vi "HandleObservationSync.vi"(8 "error in (no error)":errorcluster, 11 "S4GUI in":refnum<class "S4GUI.lvclass">) -> (0 "error out":errorcluster, 3 "S4GUI out":refnum<class "S4GUI.lvclass">)   [LabVIEW 2018, in "S4GUI.lvclass"] (continued)
            tunnel: w4130 -> [w4184 _]
            tunnel: w4124 -> [w4182 _]
            frame False {
              n1516 = case shown="0, Default" w4182 {
                selector: w4182 -> [_ w4199]
                tunnel: [w4186 w4194] -> w4183
                tunnel: w4185 -> [w4189 w4200]
                tunnel: w4184 -> [w4188 _]
                frame 0, Default {
                  n1517 = disable-structure shown="Enabled" {
                    disable-tunnel: w4188 -> [w4191 w4192]
                    disable-tunnel: [w4190 w4192] -> w4187
                    frame Disabled {
                      # "Verifica o incremento \ndo CyclesDone simultaneamente"
                      n1518 = Increment(x=w4191) -> (x+1=w4190:u32)
                    }
                    frame Enabled {
                      # "OV20241106:\nNão verifica mais o CyclesDone\nem 327 enquanto espera o ACTIVE\nem 326."
                    }
                  }
                  n1519 = Bundle By Name(cluster=w4189, "Obs_state"=w4187) -> (w4186:refnum<class "S4GUI.lvclass">)
                }
                frame 1..15 {
                  n1520 = Number To Decimal String(number=w4199) -> (decimal integer string=w4196:string)  [unwired: 1 in]
                  n1521 = Concatenate Strings("CHANNEL ERROR <", w4196, ">: Error flag TRUE - see ACS panel.  HandleObservationSync.vi - state 326.") -> (w4198:string)
                  n1522 = Bundle By Name(cluster=w4200, "Obs_state"=u32 1, "Error Msg"=w4198) -> (w4194:refnum<class "S4GUI.lvclass">)
                }
              }
            }
            frame True {
              # "ACTIVE detectado.\nIniciou aquisição..."
              n1523 = Tick Count (ms)() -> (millisecond timer value=w4201:u32)
              n1524 = local write "time307"(w4201) -> ()
              n1525 = Bundle By Name(cluster=w4204, "Obs_state"=u32 328) -> (w4203:refnum<class "S4GUI.lvclass">)
            }
          }
          n1526 = Bundle By Name(cluster=w4129, "mode EXPOSE"=w4132) -> (w4176:refnum<class "S4GUI.lvclass">)
        }
        frame 327 {
          # "T= canais receberam STOP"
          n1527 = Unbundle By Name(w4328) -> ("cyclesDone"=w4323:u32)
          n1528 = call-dynamic "Read AcquisitionA.vi"("error in (no error)"=w4361, "S4ACS_GUI in"=w4328) -> ("error out"=w4343:errorcluster, "Acquisition.lvclass"=w4344:refnum<class "Acquisition.lvclass">, "S4ACS_GUI out"=w4363:refnum<class "S4GUI.lvclass">)  [unwired: 7 in]
          n1529 = call-dynamic "Read enabled.vi"("error in (no error)"=w4343, "Server in"=w4344) -> ("error out"=w4342:errorcluster, "enabled"=w4319:bool, "Server out"=w4341:refnum<class "Acquisition.lvclass">)  [unwired: 7 in]
          n1530 = case shown="True" w4319 {
            tunnel: w4342 -> [w4517 w4534]
            tunnel: [w4518 w4532] -> w4364
            tunnel: [w4517 w4531] -> w4362
            tunnel: [0 ("State") w4527] -> w4314
            tunnel: w4341 -> [w4518 w4526]
            tunnel: w4323 -> [_ w4525]
            tunnel: [TRUE w4524] -> w4327
            tunnel: [FALSE ("stopping") w4520] -> w4310
            frame False {
            }
            frame True {
              n1531 = call-dynamic "Read Channel.vi"("error in (no error)"=w4534, "Acquisition in"=w4526) -> ("error out"=w4530:errorcluster, "Channel.lvclass"=w4529:refnum<class "Channel.lvclass">, "Acquisition out"=w4533:refnum<class "Acquisition.lvclass">)  [unwired: 7 in]
              n1532 = call-dynamic "Read CyclesDone.vi"("error in (no error)"=w4530, "Channel in"=w4529) -> ("error out"=w4522:errorcluster, "CyclesDone"=w4527:u32, "Channel out"=w4528:refnum<class "Channel.lvclass">)  [unwired: 7 in]
              n1533 = Increment(x=w4525) -> (x+1=w4519:u32)
              n1534 = Equal?(x=w4527, y=w4519) -> (x = y?=w4524:bool)
              n1535 = call-dynamic "Read stopping.vi"("error in (no error)"=w4522, "Channel in"=w4528) -> ("error out"=w4521:errorcluster, "stopping"=w4520:bool, "Channel out"=w4523:refnum<class "Channel.lvclass">)  [unwired: 7 in]
              n1536 = call-dynamic "Write Channel.vi"("error in (no error)"=w4521, "Channel.lvclass"=w4523, "Acquisition in"=w4533) -> ("error out"=w4531:errorcluster, "Acquisition out"=w4532:refnum<class "Acquisition.lvclass">)  [unwired: 7 in]
            }
          }
          n1537 = call-dynamic "Write AcquisitionA.vi"("error in (no error)"=w4362, "Acquisition.lvclass"=w4364, "S4ACS_GUI in"=w4363) -> ("error out"=w4359:errorcluster, "S4ACS_GUI out"=w4358:refnum<class "S4GUI.lvclass">)  [unwired: 7 in]
          n1538 = call "Read AcquisitionB.vi"("error in (no error)"=w4359, "S4ACS_GUI in"=w4358) -> ("error out"=w4337:errorcluster, "Acquisition.lvclass"=w4340:refnum<class "Acquisition.lvclass">, "S4ACS_GUI out"=w4360:refnum<class "S4GUI.lvclass">)  [unwired: 7 in]
          n1539 = call-dynamic "Read enabled.vi"("error in (no error)"=w4337, "Server in"=w4340) -> ("error out"=w4338:errorcluster, "enabled"=w4318:bool, "Server out"=w4339:refnum<class "Acquisition.lvclass">)  [unwired: 7 in]
          n1540 = case shown="True" w4318 {
            tunnel: w4338 -> [w4496 w4513]
            tunnel: w4339 -> [w4497 w4512]
            tunnel: [0 ("State") w4505] -> w4313
            tunnel: [w4496 w4511] -> w4357
            tunnel: [w4497 w4510] -> w4356
            tunnel: w4323 -> [_ w4504]
            tunnel: [TRUE w4503] -> w4324
            tunnel: [FALSE ("stopping") w4499] -> w4309
            frame False {
            }
            frame True {
              n1541 = call-dynamic "Read Channel.vi"("error in (no error)"=w4513, "Acquisition in"=w4512) -> ("error out"=w4508:errorcluster, "Channel.lvclass"=w4509:refnum<class "Channel.lvclass">, "Acquisition out"=w4506:refnum<class "Acquisition.lvclass">)  [unwired: 7 in]
              n1542 = call-dynamic "Read CyclesDone.vi"("error in (no error)"=w4508, "Channel in"=w4509) -> ("error out"=w4501:errorcluster, "CyclesDone"=w4505:u32, "Channel out"=w4507:refnum<class "Channel.lvclass">)  [unwired: 7 in]
              n1543 = Increment(x=w4504) -> (x+1=w4498:u32)
              n1544 = Equal?(x=w4505, y=w4498) -> (x = y?=w4503:bool)
              n1545 = call-dynamic "Read stopping.vi"("error in (no error)"=w4501, "Channel in"=w4507) -> ("error out"=w4500:errorcluster, "stopping"=w4499:bool, "Channel out"=w4502:refnum<class "Channel.lvclass">)  [unwired: 7 in]
              n1546 = call-dynamic "Write Channel.vi"("error in (no error)"=w4500, "Channel.lvclass"=w4502, "Acquisition in"=w4506) -> ("error out"=w4511:errorcluster, "Acquisition out"=w4510:refnum<class "Acquisition.lvclass">)  [unwired: 7 in]
            }
          }
          n1547 = Max & Min(x=w4314, y=w4313) -> (max(x,y)=w4326:u32)  [unwired: 1 out]
          n1548 = call "Write AcquisitionB.vi"("error in (no error)"=w4357, "Acquisition.lvclass"=w4356, "S4ACS_GUI in"=w4360) -> ("error out"=w4349:errorcluster, "S4ACS_GUI out"=w4348:refnum<class "S4GUI.lvclass">)  [unwired: 7 in]
          n1549 = call-dynamic "Read AcquisitionC.vi"("error in (no error)"=w4349, "S4ACS_GUI in"=w4348) -> ("error out"=w4334:errorcluster, "Acquisition.lvclass"=w4336:refnum<class "Acquisition.lvclass">, "S4ACS_GUI out"=w4351:refnum<class "S4GUI.lvclass">)  [unwired: 7 in]
          n1550 = call-dynamic "Read enabled.vi"("error in (no error)"=w4334, "Server in"=w4336) -> ("error out"=w4333:errorcluster, "enabled"=w4317:bool, "Server out"=w4335:refnum<class "Acquisition.lvclass">)  [unwired: 7 in]
          n1551 = case shown="True" w4317 {
            tunnel: [w4475 w4492] -> w4352
            tunnel: [w4476 w4491] -> w4350
            tunnel: w4333 -> [w4475 w4488]
            tunnel: w4335 -> [w4476 w4489]
            tunnel: [0 ("State") w4487] -> w4312
            tunnel: w4323 -> [_ w4486]
            tunnel: [TRUE w4485] -> w4322
            tunnel: [FALSE ("stopping") w4478] -> w4308
            frame False {
            }
            frame True {
              n1552 = call-dynamic "Read Channel.vi"("error in (no error)"=w4488, "Acquisition in"=w4489) -> ("error out"=w4484:errorcluster, "Channel.lvclass"=w4483:refnum<class "Channel.lvclass">, "Acquisition out"=w4490:refnum<class "Acquisition.lvclass">)  [unwired: 7 in]
              n1553 = call-dynamic "Read CyclesDone.vi"("error in (no error)"=w4484, "Channel in"=w4483) -> ("error out"=w4480:errorcluster, "CyclesDone"=w4487:u32, "Channel out"=w4482:refnum<class "Channel.lvclass">)  [unwired: 7 in]
              n1554 = Increment(x=w4486) -> (x+1=w4477:u32)
              n1555 = Equal?(x=w4487, y=w4477) -> (x = y?=w4485:bool)
              n1556 = call-dynamic "Read stopping.vi"("error in (no error)"=w4480, "Channel in"=w4482) -> ("error out"=w4479:errorcluster, "stopping"=w4478:bool, "Channel out"=w4481:refnum<class "Channel.lvclass">)  [unwired: 7 in]
              n1557 = call-dynamic "Write Channel.vi"("error in (no error)"=w4479, "Channel.lvclass"=w4481, "Acquisition in"=w4490) -> ("error out"=w4492:errorcluster, "Acquisition out"=w4491:refnum<class "Acquisition.lvclass">)  [unwired: 7 in]
            }
          }
          n1558 = call-dynamic "Write AcquisitionC.vi"("error in (no error)"=w4352, "Acquisition.lvclass"=w4350, "S4ACS_GUI in"=w4351) -> ("error out"=w4346:errorcluster, "S4ACS_GUI out"=w4347:refnum<class "S4GUI.lvclass">)  [unwired: 7 in]
          n1559 = call-dynamic "Read AcquisitionD.vi"("error in (no error)"=w4346, "S4ACS_GUI in"=w4347) -> ("error out"=w4330:errorcluster, "Acquisition.lvclass"=w4332:refnum<class "Acquisition.lvclass">, "S4ACS_GUI out"=w4353:refnum<class "S4GUI.lvclass">)  [unwired: 7 in]
          n1560 = call-dynamic "Read enabled.vi"("error in (no error)"=w4330, "Server in"=w4332) -> ("error out"=w4329:errorcluster, "enabled"=w4320:bool, "Server out"=w4331:refnum<class "Acquisition.lvclass">)  [unwired: 7 in]
          n1561 = case shown="True" w4320 {
            tunnel: [w4455 w4471] -> w4355
            tunnel: [w4454 w4470] -> w4354
            tunnel: w4331 -> [w4455 w4469]
            tunnel: w4329 -> [w4454 w4468]
            tunnel: [0 ("State") w4466] -> w4311
            tunnel: w4323 -> [_ w4465]
            tunnel: [TRUE w4464] -> w4321
            tunnel: [FALSE ("stopping") w4457] -> w4307
            frame False {
            }
            frame True {
              n1562 = call-dynamic "Read Channel.vi"("error in (no error)"=w4468, "Acquisition in"=w4469) -> ("error out"=w4463:errorcluster, "Channel.lvclass"=w4462:refnum<class "Channel.lvclass">, "Acquisition out"=w4467:refnum<class "Acquisition.lvclass">)  [unwired: 7 in]
              n1563 = call-dynamic "Read CyclesDone.vi"("error in (no error)"=w4463, "Channel in"=w4462) -> ("error out"=w4459:errorcluster, "CyclesDone"=w4466:u32, "Channel out"=w4461:refnum<class "Channel.lvclass">)  [unwired: 7 in]
              n1564 = Increment(x=w4465) -> (x+1=w4456:u32)
              n1565 = Equal?(x=w4466, y=w4456) -> (x = y?=w4464:bool)
              n1566 = call-dynamic "Read stopping.vi"("error in (no error)"=w4459, "Channel in"=w4461) -> ("error out"=w4458:errorcluster, "stopping"=w4457:bool, "Channel out"=w4460:refnum<class "Channel.lvclass">)  [unwired: 7 in]
              n1567 = call-dynamic "Write Channel.vi"("error in (no error)"=w4458, "Channel.lvclass"=w4460, "Acquisition in"=w4467) -> ("error out"=w4470:errorcluster, "Acquisition out"=w4471:refnum<class "Acquisition.lvclass">)  [unwired: 7 in]
            }
          }
          n1568 = Build Array(w4319, w4318, w4317, w4320) -> (w4316:bool[])
          n1569 = Boolean Array To Number(Boolean array=w4316) -> (number=w4315:u32)
          n1570 = Max & Min(x=w4312, y=w4311) -> (max(x,y)=w4325:u32)  [unwired: 1 out]
          n1571 = Compound Arithmetic op=AND(w4327, w4324, w4322, w4321) -> (w4306:bool)
          n1572 = case shown="15" w4315 {
            tunnel: w4314 -> [w4407 _ w4419 _ w4428 _ w4434 w4440 _ w4446 w4449 _]
            tunnel: w4311 -> [w4406 w4410 w4415 w4422 w4423 w4431 w4433 _ _ _ _ _]
            tunnel: w4313 -> [w4405 w4408 _ _ w4427 w4429 _ w4439 w4443 _ w4448 _]
            tunnel: w4312 -> [w4404 w4409 w4414 w4420 _ _ _ w4438 w4442 w4445 _ _]
            tunnel: [w4400 w4411 w4416 w4421 w4424 w4430 w4432 w4435 w4441 w4444 w4447 TRUE] -> _
            frame 15 {
              # "A,B,C,D ativos"
              n1573 = Equal?(x=w4407, y=w4405) -> (x = y?=w4403:bool)
              n1574 = Equal?(x=w4404, y=w4406) -> (x = y?=w4401:bool)
              n1575 = Equal?(x=w4405, y=w4404) -> (x = y?=w4402:bool)
              n1576 = Compound Arithmetic op=AND(w4403, w4402, w4401) -> (w4400:bool)
            }
            frame 14 {
              # "B,C e,D ativos"
              n1577 = Equal?(x=w4408, y=w4409) -> (x = y?=w4413:bool)
              n1578 = Equal?(x=w4409, y=w4410) -> (x = y?=w4412:bool)
              n1579 = Compound Arithmetic op=AND(w4413, w4412) -> (w4411:bool)
            }
            frame 13 {
              # "A,C e,D ativos"
              n1580 = Equal?(x=w4419, y=w4414) -> (x = y?=w4418:bool)
              n1581 = Equal?(x=w4414, y=w4415) -> (x = y?=w4417:bool)
              n1582 = Compound Arithmetic op=AND(w4418, w4417) -> (w4416:bool)
            }
            frame 12 {
              # "Só C e D ativos"
              n1583 = Equal?(x=w4420, y=w4422) -> (x = y?=w4421:bool)
            }
            frame 11 {
              # "A,B e,D ativos"
              n1584 = Equal?(x=w4428, y=w4427) -> (x = y?=w4426:bool)
              n1585 = Equal?(x=w4427, y=w4423) -> (x = y?=w4425:bool)
              n1586 = Compound Arithmetic op=AND(w4426, w4425) -> (w4424:bool)
            }
            frame 10 {
              # "Só B e D ativos"
              n1587 = Equal?(x=w4429, y=w4431) -> (x = y?=w4430:bool)
            }
            frame 9 {
              # "Só A e D ativos"
              n1588 = Equal?(x=w4434, y=w4433) -> (x = y?=w4432:bool)
            }
            frame 7 {
              # "A,B,C ativos"
              n1589 = Equal?(x=w4440, y=w4439) -> (x = y?=w4437:bool)
              n1590 = Equal?(x=w4439, y=w4438) -> (x = y?=w4436:bool)
              n1591 = Compound Arithmetic op=AND(w4437, w4436) -> (w4435:bool)
            }
            frame 6 {
              # "Só B e C ativos"
              n1592 = Equal?(x=w4443, y=w4442) -> (x = y?=w4441:bool)
            }
            frame 5 {
              # "Só A e C ativos"
              n1593 = Equal?(x=w4446, y=w4445) -> (x = y?=w4444:bool)
            }
            frame 3 {
              # "só A e B ativos"
              n1594 = Equal?(x=w4449, y=w4448) -> (x = y?=w4447:bool)
            }
            frame 0..2, 4, 8, Default {
              # "nenhum ou só 1  \ncanal ativo."
            }
          }
          n1595 = Max & Min(x=w4326, y=w4325) -> (max(x,y)=w4304:u32)  [unwired: 1 out]
          n1596 = Compound Arithmetic op=OR(w4310, w4309, w4308, w4307) -> (w4305:bool)
          n1597 = call-dynamic "Write AcquisitionD.vi"("error in (no error)"=w4354, "Acquisition.lvclass"=w4355, "S4ACS_GUI in"=w4353) -> ("error out"=w4345:errorcluster, "S4ACS_GUI out"=w4302:refnum<class "S4GUI.lvclass">)  [unwired: 7 in]
          n1598 = case shown="False" w4306 {
            tunnel: w4302 -> [w4367 w4388]
            tunnel: [w4373 w4387] -> w4301
            tunnel: w4305 -> [_ w4389]
            tunnel: w4304 -> [_ w4386]
            tunnel: w4303 -> [w4365 w4385]
            frame False {
              # "Aguardando iniciar exposição por 5s"
              n1599 = local read "time1"() -> (w4366:u32)
              n1600 = Tick Count (ms)() -> (millisecond timer value=w4372:u32)
              n1601 = Subtract(x=w4372, y=w4366) -> (x-y=w4369:u32)
              n1602 = To Double Precision Float(number=w4369) -> (double precision float=w4371:dbl)
              n1603 = Less?(x=5000.0 ("y"), y=w4371) -> (x < y?=w4370:bool)
              n1604 = case shown="True" w4370 {
                tunnel: w4367 -> [w4377 w4384]
                tunnel: [w4376 w4383] -> w4373
                tunnel: w4365 -> [w4375 _]
                frame False {
                  n1605 = disable-structure shown="Enabled" {
                    disable-tunnel: w4375 -> [w4379 w4380]
                    disable-tunnel: [w4378 w4380] -> w4374
                    frame Disabled {
                      # "Volta para esperar ACTIVE."
                      n1606 = Decrement(x=w4379) -> (x-1=w4378:u32)
                    }
                    frame Enabled {
                    }
                  }
                  n1607 = Bundle By Name(cluster=w4377, "Obs_state"=w4374) -> (w4376:refnum<class "S4GUI.lvclass">)
                }
                frame True {
                  n1608 = Bundle By Name(cluster=w4384, "Obs_state"=u32 1, "Error Msg"="ERROR: Init Acquisition Timeout. HandleObservationSync.vi - state 327.") -> (w4383:refnum<class "S4GUI.lvclass">)
                }
              }
            }
            frame True {
              # "STOP?"
              # "CIclo Avançou."
              n1609 = case shown="False" w4389 {
                tunnel: w4388 -> [w4393 w4399]
                tunnel: [w4392 w4398] -> w4387
                tunnel: w4386 -> [w4391 w4397]
                tunnel: w4385 -> [_ w4396]
                frame True {
                  # "STOP acionado."
                  n1610 = Bundle By Name(cluster=w4393, "Obs_state"=u32 0, "cyclesDone"=w4391) -> (w4392:refnum<class "S4GUI.lvclass">)
                }
                frame False {
                  # "Vai verificar fim dos ciclos"
                  n1611 = Increment(x=w4396) -> (x+1=w4395:u32)
                  n1612 = Increment(x=w4395) -> (x+1=w4394:u32)
                  n1613 = Bundle By Name(cluster=w4399, "Obs_state"=w4394, "cyclesDone"=w4397) -> (w4398:refnum<class "S4GUI.lvclass">)
                }
              }
            }
          }
        }
        frame 328 {
          # "T= canais receberam STOP"
          n1614 = Unbundle By Name(w4559) -> ("cyclesDone"=w4553:u32)
          n1615 = call-dynamic "Read AcquisitionA.vi"("error in (no error)"=w4595, "S4ACS_GUI in"=w4559) -> ("error out"=w4574:errorcluster, "Acquisition.lvclass"=w4575:refnum<class "Acquisition.lvclass">, "S4ACS_GUI out"=w4597:refnum<class "S4GUI.lvclass">)  [unwired: 7 in]
          n1616 = call-dynamic "Read enabled.vi"("error in (no error)"=w4574, "Server in"=w4575) -> ("error out"=w4573:errorcluster, "enabled"=w4549:bool, "Server out"=w4572:refnum<class "Acquisition.lvclass">)  [unwired: 7 in]
          n1617 = case shown="False" w4549 {
            tunnel: w4573 -> [w4746 w4763]
            tunnel: [w4747 w4761] -> w4598
            tunnel: [w4746 w4760] -> w4596
            tunnel: [0 ("State") w4756] -> w4544
            tunnel: w4572 -> [w4747 w4755]
            tunnel: w4553 -> [_ w4754]
            tunnel: [TRUE w4753] -> w4558
            tunnel: [FALSE ("stopping") w4749] -> w4540
            frame False {
            }
            frame True {
              n1618 = call-dynamic "Read Channel.vi"("error in (no error)"=w4763, "Acquisition in"=w4755) -> ("error out"=w4759:errorcluster, "Channel.lvclass"=w4758:refnum<class "Channel.lvclass">, "Acquisition out"=w4762:refnum<class "Acquisition.lvclass">)  [unwired: 7 in]
              n1619 = call-dynamic "Read CyclesDone.vi"("error in (no error)"=w4759, "Channel in"=w4758) -> ("error out"=w4751:errorcluster, "CyclesDone"=w4756:u32, "Channel out"=w4757:refnum<class "Channel.lvclass">)  [unwired: 7 in]
              n1620 = Increment(x=w4754) -> (x+1=w4748:u32)
              n1621 = Equal?(x=w4756, y=w4748) -> (x = y?=w4753:bool)
              n1622 = call-dynamic "Read stopping.vi"("error in (no error)"=w4751, "Channel in"=w4757) -> ("error out"=w4750:errorcluster, "stopping"=w4749:bool, "Channel out"=w4752:refnum<class "Channel.lvclass">)  [unwired: 7 in]
              n1623 = call-dynamic "Write Channel.vi"("error in (no error)"=w4750, "Channel.lvclass"=w4752, "Acquisition in"=w4762) -> ("error out"=w4760:errorcluster, "Acquisition out"=w4761:refnum<class "Acquisition.lvclass">)  [unwired: 7 in]
            }
          }
          n1624 = call-dynamic "Write AcquisitionA.vi"("error in (no error)"=w4596, "Acquisition.lvclass"=w4598, "S4ACS_GUI in"=w4597) -> ("error out"=w4591:errorcluster, "S4ACS_GUI out"=w4590:refnum<class "S4GUI.lvclass">)  [unwired: 7 in]
          n1625 = call "Read AcquisitionB.vi"("error in (no error)"=w4591, "S4ACS_GUI in"=w4590) -> ("error out"=w4568:errorcluster, "Acquisition.lvclass"=w4571:refnum<class "Acquisition.lvclass">, "S4ACS_GUI out"=w4592:refnum<class "S4GUI.lvclass">)  [unwired: 7 in]
          n1626 = call-dynamic "Read enabled.vi"("error in (no error)"=w4568, "Server in"=w4571) -> ("error out"=w4569:errorcluster, "enabled"=w4548:bool, "Server out"=w4570:refnum<class "Acquisition.lvclass">)  [unwired: 7 in]
          n1627 = case shown="True" w4548 {
            tunnel: w4569 -> [w4725 w4742]
            tunnel: w4570 -> [w4726 w4741]
            tunnel: [0 ("State") w4734] -> w4543
            tunnel: [w4725 w4740] -> w4589
            tunnel: [w4726 w4739] -> w4588
            tunnel: w4553 -> [_ w4733]
            tunnel: [TRUE w4732] -> w4554
            tunnel: [FALSE ("stopping") w4728] -> w4539
            frame False {
            }
            frame True {
              n1628 = call-dynamic "Read Channel.vi"("error in (no error)"=w4742, "Acquisition in"=w4741) -> ("error out"=w4737:errorcluster, "Channel.lvclass"=w4738:refnum<class "Channel.lvclass">, "Acquisition out"=w4735:refnum<class "Acquisition.lvclass">)  [unwired: 7 in]
              n1629 = call-dynamic "Read CyclesDone.vi"("error in (no error)"=w4737, "Channel in"=w4738) -> ("error out"=w4730:errorcluster, "CyclesDone"=w4734:u32, "Channel out"=w4736:refnum<class "Channel.lvclass">)  [unwired: 7 in]
              n1630 = Increment(x=w4733) -> (x+1=w4727:u32)
              n1631 = Equal?(x=w4734, y=w4727) -> (x = y?=w4732:bool)
              n1632 = call-dynamic "Read stopping.vi"("error in (no error)"=w4730, "Channel in"=w4736) -> ("error out"=w4729:errorcluster, "stopping"=w4728:bool, "Channel out"=w4731:refnum<class "Channel.lvclass">)  [unwired: 7 in]
              n1633 = call-dynamic "Write Channel.vi"("error in (no error)"=w4729, "Channel.lvclass"=w4731, "Acquisition in"=w4735) -> ("error out"=w4740:errorcluster, "Acquisition out"=w4739:refnum<class "Acquisition.lvclass">)  [unwired: 7 in]
            }
          }
          n1634 = Max & Min(x=w4544, y=w4543) -> (max(x,y)=w4557:u32)  [unwired: 1 out]
          n1635 = call "Write AcquisitionB.vi"("error in (no error)"=w4589, "Acquisition.lvclass"=w4588, "S4ACS_GUI in"=w4592) -> ("error out"=w4581:errorcluster, "S4ACS_GUI out"=w4580:refnum<class "S4GUI.lvclass">)  [unwired: 7 in]
          n1636 = call-dynamic "Read AcquisitionC.vi"("error in (no error)"=w4581, "S4ACS_GUI in"=w4580) -> ("error out"=w4565:errorcluster, "Acquisition.lvclass"=w4567:refnum<class "Acquisition.lvclass">, "S4ACS_GUI out"=w4583:refnum<class "S4GUI.lvclass">)  [unwired: 7 in]
          n1637 = call-dynamic "Read enabled.vi"("error in (no error)"=w4565, "Server in"=w4567) -> ("error out"=w4564:errorcluster, "enabled"=w4547:bool, "Server out"=w4566:refnum<class "Acquisition.lvclass">)  [unwired: 7 in]
          n1638 = case shown="False" w4547 {
            tunnel: [w4704 w4721] -> w4584
            tunnel: [w4705 w4720] -> w4582
            tunnel: w4564 -> [w4704 w4717]
            tunnel: w4566 -> [w4705 w4718]
            tunnel: [0 ("State") w4716] -> w4542
            tunnel: w4553 -> [_ w4715]
            tunnel: [TRUE w4714] -> w4552
            tunnel: [FALSE ("stopping") w4707] -> w4538
            frame False {
            }
            frame True {
              n1639 = call-dynamic "Read Channel.vi"("error in (no error)"=w4717, "Acquisition in"=w4718) -> ("error out"=w4713:errorcluster, "Channel.lvclass"=w4712:refnum<class "Channel.lvclass">, "Acquisition out"=w4719:refnum<class "Acquisition.lvclass">)  [unwired: 7 in]
              n1640 = call-dynamic "Read CyclesDone.vi"("error in (no error)"=w4713, "Channel in"=w4712) -> ("error out"=w4709:errorcluster, "CyclesDone"=w4716:u32, "Channel out"=w4711:refnum<class "Channel.lvclass">)  [unwired: 7 in]
              n1641 = Increment(x=w4715) -> (x+1=w4706:u32)
              n1642 = Equal?(x=w4716, y=w4706) -> (x = y?=w4714:bool)
              n1643 = call-dynamic "Read stopping.vi"("error in (no error)"=w4709, "Channel in"=w4711) -> ("error out"=w4708:errorcluster, "stopping"=w4707:bool, "Channel out"=w4710:refnum<class "Channel.lvclass">)  [unwired: 7 in]
              n1644 = call-dynamic "Write Channel.vi"("error in (no error)"=w4708, "Channel.lvclass"=w4710, "Acquisition in"=w4719) -> ("error out"=w4721:errorcluster, "Acquisition out"=w4720:refnum<class "Acquisition.lvclass">)  [unwired: 7 in]
            }
          }
          n1645 = call-dynamic "Write AcquisitionC.vi"("error in (no error)"=w4584, "Acquisition.lvclass"=w4582, "S4ACS_GUI in"=w4583) -> ("error out"=w4578:errorcluster, "S4ACS_GUI out"=w4579:refnum<class "S4GUI.lvclass">)  [unwired: 7 in]
          n1646 = call-dynamic "Read AcquisitionD.vi"("error in (no error)"=w4578, "S4ACS_GUI in"=w4579) -> ("error out"=w4561:errorcluster, "Acquisition.lvclass"=w4563:refnum<class "Acquisition.lvclass">, "S4ACS_GUI out"=w4585:refnum<class "S4GUI.lvclass">)  [unwired: 7 in]
          n1647 = call-dynamic "Read enabled.vi"("error in (no error)"=w4561, "Server in"=w4563) -> ("error out"=w4560:errorcluster, "enabled"=w4550:bool, "Server out"=w4562:refnum<class "Acquisition.lvclass">)  [unwired: 7 in]
          n1648 = case shown="True" w4550 {
            tunnel: [w4684 w4700] -> w4587
            tunnel: [w4683 w4699] -> w4586
            tunnel: w4562 -> [w4684 w4698]
            tunnel: w4560 -> [w4683 w4697]
            tunnel: [0 ("State") w4695] -> w4541
            tunnel: w4553 -> [_ w4694]
            tunnel: [TRUE w4693] -> w4551
            tunnel: [FALSE ("stopping") w4686] -> w4537
            frame False {
            }
            frame True {
              n1649 = call-dynamic "Read Channel.vi"("error in (no error)"=w4697, "Acquisition in"=w4698) -> ("error out"=w4692:errorcluster, "Channel.lvclass"=w4691:refnum<class "Channel.lvclass">, "Acquisition out"=w4696:refnum<class "Acquisition.lvclass">)  [unwired: 7 in]
              n1650 = call-dynamic "Read CyclesDone.vi"("error in (no error)"=w4692, "Channel in"=w4691) -> ("error out"=w4688:errorcluster, "CyclesDone"=w4695:u32, "Channel out"=w4690:refnum<class "Channel.lvclass">)  [unwired: 7 in]
              n1651 = Increment(x=w4694) -> (x+1=w4685:u32)
              n1652 = Equal?(x=w4695, y=w4685) -> (x = y?=w4693:bool)
              n1653 = call-dynamic "Read stopping.vi"("error in (no error)"=w4688, "Channel in"=w4690) -> ("error out"=w4687:errorcluster, "stopping"=w4686:bool, "Channel out"=w4689:refnum<class "Channel.lvclass">)  [unwired: 7 in]
              n1654 = call-dynamic "Write Channel.vi"("error in (no error)"=w4687, "Channel.lvclass"=w4689, "Acquisition in"=w4696) -> ("error out"=w4699:errorcluster, "Acquisition out"=w4700:refnum<class "Acquisition.lvclass">)  [unwired: 7 in]
            }
          }
          n1655 = Build Array(w4549, w4548, w4547, w4550) -> (w4546:bool[])
          n1656 = Boolean Array To Number(Boolean array=w4546) -> (number=w4545:u32)
          n1657 = Max & Min(x=w4542, y=w4541) -> (max(x,y)=w4556:u32)  [unwired: 1 out]
          n1658 = Compound Arithmetic op=AND(w4558, w4554, w4552, w4551) -> (w4535:bool)
          n1659 = case shown="15" w4545 {
            tunnel: w4544 -> [w4606 _ w4618 _ w4627 _ w4633 w4639 _ w4645 w4648 _]
            tunnel: w4541 -> [w4605 w4609 w4614 w4621 w4622 w4630 w4632 _ _ _ _ _]
            tunnel: w4543 -> [w4604 w4607 _ _ w4626 w4628 _ w4638 w4642 _ w4647 _]
            tunnel: w4542 -> [w4603 w4608 w4613 w4619 _ _ _ w4637 w4641 w4644 _ _]
            tunnel: [w4599 w4610 w4615 w4620 w4623 w4629 w4631 w4634 w4640 w4643 w4646 TRUE] -> _
            frame 15 {
              # "A,B,C,D ativos"
              n1660 = Equal?(x=w4606, y=w4604) -> (x = y?=w4602:bool)
              n1661 = Equal?(x=w4603, y=w4605) -> (x = y?=w4600:bool)
              n1662 = Equal?(x=w4604, y=w4603) -> (x = y?=w4601:bool)
              n1663 = Compound Arithmetic op=AND(w4602, w4601, w4600) -> (w4599:bool)
            }
            frame 14 {
              # "B,C e,D ativos"
              n1664 = Equal?(x=w4607, y=w4608) -> (x = y?=w4612:bool)
              n1665 = Equal?(x=w4608, y=w4609) -> (x = y?=w4611:bool)
              n1666 = Compound Arithmetic op=AND(w4612, w4611) -> (w4610:bool)
            }
            frame 13 {
              # "A,C e,D ativos"
              n1667 = Equal?(x=w4618, y=w4613) -> (x = y?=w4617:bool)
              n1668 = Equal?(x=w4613, y=w4614) -> (x = y?=w4616:bool)
              n1669 = Compound Arithmetic op=AND(w4617, w4616) -> (w4615:bool)
            }
            frame 12 {
              # "Só C e D ativos"
              n1670 = Equal?(x=w4619, y=w4621) -> (x = y?=w4620:bool)
            }
            frame 11 {
              # "A,B e,D ativos"
              n1671 = Equal?(x=w4627, y=w4626) -> (x = y?=w4625:bool)
              n1672 = Equal?(x=w4626, y=w4622) -> (x = y?=w4624:bool)
              n1673 = Compound Arithmetic op=AND(w4625, w4624) -> (w4623:bool)
            }
            frame 10 {
              # "Só B e D ativos"
              n1674 = Equal?(x=w4628, y=w4630) -> (x = y?=w4629:bool)
            }
            frame 9 {
              # "Só A e D ativos"
              n1675 = Equal?(x=w4633, y=w4632) -> (x = y?=w4631:bool)
            }
            frame 7 {
              # "A,B,C ativos"
              n1676 = Equal?(x=w4639, y=w4638) -> (x = y?=w4636:bool)
              n1677 = Equal?(x=w4638, y=w4637) -> (x = y?=w4635:bool)
              n1678 = Compound Arithmetic op=AND(w4636, w4635) -> (w4634:bool)
            }
            frame 6 {
              # "Só B e C ativos"
              n1679 = Equal?(x=w4642, y=w4641) -> (x = y?=w4640:bool)
            }
            frame 5 {
              # "Só A e C ativos"
              n1680 = Equal?(x=w4645, y=w4644) -> (x = y?=w4643:bool)
            }
            frame 3 {
              # "só A e B ativos"
              n1681 = Equal?(x=w4648, y=w4647) -> (x = y?=w4646:bool)
            }
            frame 0..2, 4, 8, Default {
              # "nenhum ou só 1  \ncanal ativo."
            }
          }
          n1682 = Max & Min(x=w4557, y=w4556) -> (max(x,y)=w4555:u32)  [unwired: 1 out]
          n1683 = Compound Arithmetic op=OR(w4540, w4539, w4538, w4537) -> (w4536:bool)
          n1684 = call-dynamic "Write AcquisitionD.vi"("error in (no error)"=w4586, "Acquisition.lvclass"=w4587, "S4ACS_GUI in"=w4585) -> ("error out"=w4576:errorcluster, "S4ACS_GUI out"=w4577:refnum<class "S4GUI.lvclass">)  [unwired: 7 in]
          n1685 = case shown="False" w4535 {
            tunnel: w4577 -> [w4660 w4670]
            tunnel: [w4659 w4669] -> w4594
            tunnel: w4593 -> [_ w4668]
            tunnel: w4555 -> [_ w4667]
            tunnel: w4536 -> [_ w4666]
            frame False {
              # "Aguardando avanço do ciclo."
              n1686 = local read "time307"() -> (w4650:u32)
              n1687 = Tick Count (ms)() -> (millisecond timer value=w4658:u32)
              n1688 = Subtract(x=w4658, y=w4650) -> (x-y=w4655:u32)
              n1689 = call-dynamic "GetGreatestCube.vi"("S4GUI in"=w4660) -> ("S4GUI out"=w4651:refnum<class "S4GUI.lvclass">, "greatest (ms)"=w4653:dbl)  [unwired: 8 in, 1 out]
              n1690 = To Double Precision Float(number=w4655) -> (double precision float=w4657:dbl)
              n1691 = Add(x=5000.0 ("y"), y=w4653) -> (x+y=w4652:dbl)
              n1692 = Less?(x=w4652, y=w4657) -> (x < y?=w4656:bool)
              n1693 = case shown="False" w4656 {
                tunnel: w4651 -> [w4661 w4665]
                tunnel: [w4661 w4664] -> w4659
                frame False {
                }
                frame True {
                  n1694 = Bundle By Name(cluster=w4665, "Obs_state"=u32 1, "Error Msg"="ERROR: Acquisition Timeout. HandleObservationSync.vi - state 328.") -> (w4664:refnum<class "S4GUI.lvclass">)
                }
              }
            }
            frame True {
              # "Ciclo avançou."
              # "STOP?"
              n1695 = case shown="False" w4666 {
                tunnel: w4670 -> [w4674 w4679]
                tunnel: [w4673 w4678] -> w4669
                tunnel: w4668 -> [_ w4676]
                tunnel: w4667 -> [w4672 w4675]
                frame True {
                  n1696 = Bundle By Name(cluster=w4674, "Obs_state"=u32 0, "cyclesDone"=w4672) -> (w4673:refnum<class "S4GUI.lvclass">)
                }
                frame False {
                  n1697 = Increment(x=w4676) -> (x+1=w4677:u32)
                  n1698 = Bundle By Name(cluster=w4679, "Obs_state"=w4677, "cyclesDone"=w4675) -> (w4678:refnum<class "S4GUI.lvclass">)
                }
              }
            }
          }
        }
        frame 329 {
          n1699 = disable-structure shown="Enabled" {
            disable-tunnel: w4768 -> [w4782 w4788]
            disable-tunnel: w4767 -> [w4781 w4795]
            disable-tunnel: [w4780 w4795] -> w4766
            disable-tunnel: [w4778 w4796] -> w4765
            disable-tunnel: w4764 -> [_ w4789]
            frame Disabled {
              n1700 = call-dynamic "Read ciclos.vi"("error in (no error)"=w4781, "S4ACS_GUI in"=w4782) -> ("error out"=w4770:errorcluster, "ciclos"=w4775:u32, "S4ACS_GUI out"=w4783:refnum<class "S4GUI.lvclass">)  [unwired: 7 in]
              n1701 = Decrement(x=w4775) -> (x-1=w4769:u32)
              n1702 = Greater Than 0?(x=w4769) -> (x > 0?=w4776:bool)
              n1703 = case shown="False" w4776 {
                selector: w4776 -> [w4785 w4787]
                tunnel: w4769 -> [_ w4786]
                tunnel: [w4785 w4787] -> w4774
                tunnel: [u32 0 w4786] -> w4771
                frame False {
                }
                frame True {
                }
              }
              n1704 = Select(t=u32 323, s=w4774, f=u32 0) -> (s? t:f=w4777:u32)
              n1705 = call-dynamic "Write ciclos.vi"("error in (no error)"=w4770, "ciclos"=w4771, "S4ACS_GUI in"=w4783) -> ("error out"=w4780:errorcluster, "S4ACS_GUI out"=w4779:refnum<class "S4GUI.lvclass">)  [unwired: 7 in]
              n1706 = Bundle By Name(cluster=w4779, "Obs_state"=w4777) -> (w4778:refnum<class "S4GUI.lvclass">)
            }
            frame Enabled {
              n1707 = Unbundle By Name(w4788) -> ("TotalCiclos"=w4798:u32, "cyclesDone"=w4797:u32)
              n1708 = Subtract(x=w4798, y=w4797) -> (x-y=w4791:u32)
              n1709 = Greater Than 0?(x=w4791) -> (x > 0?=w4794:bool)
              n1710 = disable-structure shown="Enabled" {
                disable-tunnel: [w4800 u32 325 ("t")] -> w4790
                disable-tunnel: w4789 -> [w4799 _]
                frame Disabled {
                  n1711 = Increment(x=w4799) -> (x+1=w4800:u32)
                }
                frame Enabled {
                }
              }
              n1712 = Select(t=w4790, s=w4794, f=u32 0) -> (s? t:f=w4793:u32)
              n1713 = Bundle By Name(cluster=w4788, "ciclos"=w4791, "Obs_state"=w4793) -> (w4796:refnum<class "S4GUI.lvclass">)
            }
          }
        }
        frame 350 {
          n1714 = flat-sequence {
            tunnel: w4803 -> [w4843]
            tunnel: [w4843] -> w4802
            frame #0 {
              n1715 = Tick Count (ms)() -> (millisecond timer value=→"timer350":u32)
            }
          }
          n1716 = call "Read Instrument.lvclass.vi"("error in (no error)"=w4802, "S4ACS_GUI in"=w4838) -> ("error out"=w4841:errorcluster, "Instrument.lvclass"=w4842:refnum<class "Instrument.lvclass">, "S4ACS_GUI out"=w4839:refnum<class "S4GUI.lvclass">)  [unwired: 7 in]
          n1717 = call "Read WPROT.vi"("error in (no error)"=w4841, "Instrument in"=w4842) -> ("error out"=w4831:errorcluster, "Opt_Selector.lvclass"=w4832:refnum<class "Opt_Selector.lvclass">, "Instrument out"=w4840:refnum<class "Instrument.lvclass">)  [unwired: 7 in]
          n1718 = call-dynamic "getTargetPos.vi"("error in (no error)"=w4831, "Opt_Selector in"=w4832) -> ("error out"=w4830:errorcluster, "Target Pos"=w4810:u16, "Opt_Selector out"=w4829:refnum<class "Opt_Selector.lvclass">)  [unwired: 7 in]
          n1719 = Build Array(-1.0 ("element"), 0.0 ("element"), 22.5 ("element"), 45.0 ("element"), 67.5 ("element"), 90.0 ("element"), 112.5 ("element"), 135.0 ("element"), 157.5 ("element"), 180.0 ("element"), 202.5 ("element"), 225.0 ("element"), 247.5 ("element"), 270.0 ("element"), 292.5 ("element"), 315.0 ("element"), 337.5 ("element")) -> (w4822:dbl[])
          n1720 = Index Array(array=w4822, index=w4810) -> (element=w4809:dbl)
          n1721 = case shown="0, Default" w4810 {
            selector: w4810 -> [_ w4872]
            tunnel: w4840 -> [w4852 w4860]
            tunnel: [w4852 w4860] -> w4805
            tunnel: [w4849 w4859] -> w4804
            tunnel: w4835 -> [_ w4874]
            tunnel: [u32 352 w4873] -> w4834
            tunnel: w4830 -> [w4850 w4868]
            tunnel: w4829 -> [w4851 w4867]
            tunnel: w4809 -> [_ w4862]
            tunnel: [w4847 w4861] -> w4806
            frame 0, Default {
              # "Terminou uma sequência.\nRecupera as posições em SEQ e desvia para 311 para verificar se há mais ciclos."
              # "Recupera a sequencia anterior para o caso \nde repetição da sequencia (sem precisar clicar \nnas posicoes desejadas novamente)."
              n1722 = call-dynamic "Read sequencia_ant.vi"("error in (no error)"=w4850, "Opt_Selector in"=w4851) -> ("error out"=w4846:errorcluster, "sequencia_ant"=w4845:u16, "Opt_Selector out"=w4848:refnum<class "Opt_Selector.lvclass">)  [unwired: 7 in]
              n1723 = call-dynamic "Write sequencia.vi"("error in (no error)"=w4846, "sequencia"=w4845, "Opt_Selector in"=w4848) -> ("error out"=w4849:errorcluster, "Opt_Selector out"=w4847:refnum<class "Opt_Selector.lvclass">)  [unwired: 7 in]
            }
            frame 1..16 {
              # "Espera até 40 x 0.25s (= 10s) para\nmecanismo entrar em READY"
              n1724 = Number To Decimal String(number=w4872) -> (decimal integer string=w4871:string)  [unwired: 1 in]
              n1725 = Concatenate Strings("WP" ("string"), w4871) -> (w4869:string)
              n1726 = call "Write target name.vi"("error in (no error)"=w4868, "target name"=w4869, "Optics in"=w4867) -> ("error out"=w4865:errorcluster, "Optics out"=w4866:refnum<class "Opt_Selector.lvclass">)  [unwired: 7 in]
              n1727 = call "Write target.vi"("error in (no error)"=w4865, "target"=w4862, "Optics in"=w4866) -> ("error out"=w4864:errorcluster, "Optics out"=w4863:refnum<class "Opt_Selector.lvclass">)  [unwired: 7 in]
              n1728 = call-dynamic "Read State Machine.vi"("error in (no error)"=w4864, "Device in"=w4863) -> ("error out"=w4876:errorcluster, "State Machine.lvclass"=w4878:refnum<class "State Machine.lvclass">, "Device out"=w4875:refnum<class "Opt_Selector.lvclass">)  [unwired: 7 in]
              n1729 = Increment(x=w4874) -> (x+1=w4873:u32)
              n1730 = call "Next State.vi"("error in (no error)"=w4876, "New_State"=1, "State Machine in"=w4878) -> ("error out"=w4856:errorcluster, "State Machine out"=w4858:refnum<class "State Machine.lvclass">)  [unwired: 7 in]
              n1731 = call-dynamic "Write Timer.vi"("error in (no error)"=w4856, "Timer"=u32 40, "State Machine in"=w4858) -> ("error out"=w4855:errorcluster, "State Machine out"=w4857:refnum<class "State Machine.lvclass">)  [unwired: 7 in]
              n1732 = call-dynamic "Write State Machine.vi"("error in (no error)"=w4855, "State Machine.lvclass"=w4857, "Device in"=w4875) -> ("error out"=w4859:errorcluster, "Device out"=w4861:refnum<class "Opt_Selector.lvclass">)  [unwired: 7 in]
            }
          }
          n1733 = call "Write WPROT.vi"("error in (no error)"=w4804, "Opt_Selector.lvclass"=w4806, "Instrument in"=w4805) -> ("error out"=w4808:errorcluster, "Instrument out"=w4807:refnum<class "Instrument.lvclass">)  [unwired: 7 in]
          n1734 = call "Write Instrument.lvclass.vi"("error in (no error)"=w4808, "Instrument.lvclass"=w4807, "S4ACS_GUI in"=w4839) -> ("error out"=w4837:errorcluster, "S4ACS_GUI out"=w4836:refnum<class "S4GUI.lvclass">)  [unwired: 7 in]
          n1735 = Bundle By Name(cluster=w4836, "Obs_state"=w4834) -> (w4833:refnum<class "S4GUI.lvclass">)
        }
        frame 351 {
          # "Espera terminar o movimento da lamina para disparar a aquisição\ndos canais ativos.\n\nOV 20230424: Não precisa mais atualizar o valor de WPPOS com o\ncomando WRITE_HEADER porque o ACS já recebeu a sequência de\nposições da lâmina."
          n1736 = flat-sequence {
            tunnel: w4889 -> [w4908]
            tunnel: [w4908] -> w4888
            frame #0 {
              n1737 = Tick Count (ms)() -> (millisecond timer value=w4907:u32)
              "timer351" <- w4907
              n1738 = local read "time1"() -> (w4906:u32)
              n1739 = Subtract(x=w4907, y=w4906) -> (x-y=→"delay wp 2":u32)
            }
          }
          n1740 = call "Read Instrument.lvclass.vi"("error in (no error)"=w4888, "S4ACS_GUI in"=w4898) -> ("error out"=w4903:errorcluster, "Instrument.lvclass"=w4904:refnum<class "Instrument.lvclass">, "S4ACS_GUI out"=w4900:refnum<class "S4GUI.lvclass">)  [unwired: 7 in]
          n1741 = call "Read WPROT.vi"("error in (no error)"=w4903, "Instrument in"=w4904) -> ("error out"=w4895:errorcluster, "Opt_Selector.lvclass"=w4894:refnum<class "Opt_Selector.lvclass">, "Instrument out"=w4902:refnum<class "Instrument.lvclass">)  [unwired: 7 in]
          n1742 = call-dynamic "Read State Machine.vi"("error in (no error)"=w4895, "Device in"=w4894) -> ("error out"=w4896:errorcluster, "State Machine.lvclass"=w4897:refnum<class "State Machine.lvclass">, "Device out"=w4892:refnum<class "Opt_Selector.lvclass">)  [unwired: 7 in]
          n1743 = call-dynamic "Read State.vi"("error in (no error)"=w4896, "State Machine in"=w4897) -> ("error out"=w4886:errorcluster, "State"=w4890:i32, "State Machine out"=w4887:refnum<class "State Machine.lvclass">)  [unwired: 7 in]
          n1744 = Equal To 0?(x=w4890) -> (x = 0?=w4881:bool)
          n1745 = call-dynamic "Write State Machine.vi"("error in (no error)"=w4886, "State Machine.lvclass"=w4887, "Device in"=w4892) -> ("error out"=w4891:errorcluster, "Device out"=w4893:refnum<class "Opt_Selector.lvclass">)  [unwired: 7 in]
          n1746 = call "Write WPROT.vi"("error in (no error)"=w4891, "Opt_Selector.lvclass"=w4893, "Instrument in"=w4902) -> ("error out"=w4899:errorcluster, "Instrument out"=w4901:refnum<class "Instrument.lvclass">)  [unwired: 7 in]
          n1747 = call "Write Instrument.lvclass.vi"("error in (no error)"=w4899, "Instrument.lvclass"=w4901, "S4ACS_GUI in"=w4900) -> ("error out"=w4879:errorcluster, "S4ACS_GUI out"=w4882:refnum<class "S4GUI.lvclass">)  [unwired: 7 in]
          n1748 = Select(t=u32 350, s=w4881, f=w4880) -> (s? t:f=w4885:u32)
          n1749 = Bundle By Name(cluster=w4882, "Obs_state"=w4885) -> (w4883:refnum<class "S4GUI.lvclass">)
        }
        frame 352 {
          n1750 = disable-structure shown="Enabled" {
            disable-tunnel: w4912 -> [w4926 w4939]
            disable-tunnel: w4911 -> [w4925 w4937]
            disable-tunnel: [w4924 w4937] -> w4910
            disable-tunnel: [w4922 w4938] -> w4909
            frame Disabled {
              n1751 = call-dynamic "Read ciclos.vi"("error in (no error)"=w4925, "S4ACS_GUI in"=w4926) -> ("error out"=w4914:errorcluster, "ciclos"=w4919:u32, "S4ACS_GUI out"=w4927:refnum<class "S4GUI.lvclass">)  [unwired: 7 in]
              n1752 = Decrement(x=w4919) -> (x-1=w4913:u32)
              n1753 = Greater Than 0?(x=w4913) -> (x > 0?=w4920:bool)
              n1754 = case shown="False" w4920 {
                selector: w4920 -> [w4929 w4931]
                tunnel: w4913 -> [_ w4930]
                tunnel: [w4929 w4931] -> w4918
                tunnel: [u32 0 w4930] -> w4915
                frame False {
                }
                frame True {
                }
              }
              n1755 = Select(t=u32 323, s=w4918, f=u32 0) -> (s? t:f=w4921:u32)
              n1756 = call-dynamic "Write ciclos.vi"("error in (no error)"=w4914, "ciclos"=w4915, "S4ACS_GUI in"=w4927) -> ("error out"=w4924:errorcluster, "S4ACS_GUI out"=w4923:refnum<class "S4GUI.lvclass">)  [unwired: 7 in]
              n1757 = Bundle By Name(cluster=w4923, "Obs_state"=w4921) -> (w4922:refnum<class "S4GUI.lvclass">)
            }
            frame Enabled {
              n1758 = Unbundle By Name(w4939) -> ("cycles wprot"=w4940:u32)
              n1759 = Decrement(x=w4940) -> (x-1=w4932:u32)
              n1760 = Greater Than 0?(x=w4932) -> (x > 0?=w4936:bool)
              n1761 = Select(t=u32 350, s=w4936, f=u32 0) -> (s? t:f=w4935:u32)
              n1762 = Bundle By Name(cluster=w4939, "Obs_state"=w4935, "cycles wprot"=w4932) -> (w4938:refnum<class "S4GUI.lvclass">)
            }
          }
        }
        frame 360 {
          w4941 = u32 0 ("cyclesDone")
          # "Inicia o Ticks com\nvalor do relogio atual"
          # "Espera até 40 x 0.25s (= 10s) para\nmecanismo entrar em READY"
          # "Busca próximo valor de foco..."
          n1763 = flat-sequence {
            tunnel: w4958 -> [w4973]
            tunnel: [w4973] -> w4957
            frame #0 {
              n1764 = Tick Count (ms)() -> (millisecond timer value=→"time7":u32)
            }
          }
          n1765 = call-dynamic "Read TelFocus.lvclass.vi"("error in (no error)"=w4957, "S4GUI in"=w4969) -> ("error out"=w4971:errorcluster, "TelFocus.lvclass"=w4972:refnum<class "TelFocus.lvclass">, "S4GUI out"=w4970:refnum<class "S4GUI.lvclass">)  [unwired: 7 in]
          n1766 = call-dynamic "GetNextFocus.vi"("error in (no error)"=w4971, "TelFocus in"=w4972) -> ("error out"=w4955:errorcluster, "TelFocus out"=w4956:refnum<class "TelFocus.lvclass">)  [unwired: 8 in]
          n1767 = call-dynamic "Read SecMirror.lvclass.vi"("error in (no error)"=w4955, "TelFocus in"=w4956) -> ("error out"=w4942:errorcluster, "SecMirror.lvclass"=w4943:refnum<class "SecMirror.lvclass">, "TelFocus out"=w4960:refnum<class "TelFocus.lvclass">)  [unwired: 7 in]
          n1768 = call-dynamic "Read State Machine.vi"("error in (no error)"=w4942, "Device in"=w4943) -> ("error out"=w4952:errorcluster, "State Machine.lvclass"=w4954:refnum<class "State Machine.lvclass">, "Device out"=w4951:refnum<class "SecMirror.lvclass">)  [unwired: 7 in]
          n1769 = call "Next State.vi"("error in (no error)"=w4952, "New_State"=1, "State Machine in"=w4954) -> ("error out"=w4949:errorcluster, "State Machine out"=w4950:refnum<class "State Machine.lvclass">)  [unwired: 7 in]
          n1770 = call-dynamic "Write Timer.vi"("error in (no error)"=w4949, "Timer"=u32 40, "State Machine in"=w4950) -> ("error out"=w4946:errorcluster, "State Machine out"=w4947:refnum<class "State Machine.lvclass">)  [unwired: 7 in]
          n1771 = call-dynamic "Init Ticks2.vi"("error in (no error)"=w4946, "State Machine in"=w4947) -> ("error out"=w4945:errorcluster, "State Machine out"=w4944:refnum<class "State Machine.lvclass">)  [unwired: 8 in]
          n1772 = call-dynamic "Write State Machine.vi"("error in (no error)"=w4945, "State Machine.lvclass"=w4944, "Device in"=w4951) -> ("error out"=w4959:errorcluster, "Device out"=w4961:refnum<class "SecMirror.lvclass">)  [unwired: 7 in]
          n1773 = call-dynamic "Write SecMirror.lvclass.vi"("error in (no error)"=w4959, "SecMirror.lvclass"=w4961, "TelFocus in"=w4960) -> ("error out"=w4963:errorcluster, "TelFocus out"=w4962:refnum<class "TelFocus.lvclass">)  [unwired: 7 in]
          n1774 = call-dynamic "Write TelFocus.lvclass.vi"("error in (no error)"=w4963, "TelFocus.lvclass"=w4962, "S4GUI in"=w4970) -> ("error out"=w4968:errorcluster, "S4GUI out"=w4967:refnum<class "S4GUI.lvclass">)  [unwired: 7 in]
          n1775 = Increment(x=w4966) -> (x+1=w4965:u32)
          n1776 = Bundle By Name(cluster=w4967, "Obs_state"=w4965, "cyclesDone"=w4941, "sequesDone"=w4941) -> (w4964:refnum<class "S4GUI.lvclass">)
        }
        frame 361 {
          # "90: estado de erro."
          # "Timeout= 25s + distancia do target (cada 1000um=1s)"
          # "Espera terminar o movimento do foco do 2ndario para \ndisparar a aquisição do canal."
          n1777 = flat-sequence {
            tunnel: w5013 -> [w5035]
            tunnel: [w5035] -> w5012
            frame #0 {
              n1778 = Tick Count (ms)() -> (millisecond timer value=w5034:u32)
              "time 8" <- w5034
              n1779 = local read "time1"() -> (w5033:u32)
              n1780 = Subtract(x=w5034, y=w5033) -> (x-y=→"delay 78":u32)
            }
          }
          n1781 = call-dynamic "Read TelFocus.lvclass.vi"("error in (no error)"=w5012, "S4GUI in"=w5017) -> ("error out"=w5022:errorcluster, "TelFocus.lvclass"=w5023:refnum<class "TelFocus.lvclass">, "S4GUI out"=w5019:refnum<class "S4GUI.lvclass">)  [unwired: 7 in]
          n1782 = call-dynamic "Read SecMirror.lvclass.vi"("error in (no error)"=w5022, "TelFocus in"=w5023) -> ("error out"=w4991:errorcluster, "SecMirror.lvclass"=w4994:refnum<class "SecMirror.lvclass">, "TelFocus out"=w5021:refnum<class "TelFocus.lvclass">)  [unwired: 7 in]
          n1783 = call-dynamic "Read position.vi"("error in (no error)"=w4991, "SecMirror in"=w4994) -> ("error out"=w4990:errorcluster, "position"=w4987:i32, "SecMirror out"=w4993:refnum<class "SecMirror.lvclass">)  [unwired: 7 in]
          n1784 = call-dynamic "Read target.vi"("error in (no error)"=w4990, "SecMirror in"=w4993) -> ("error out"=w4989:errorcluster, "target"=w4988:i32, "SecMirror out"=w4992:refnum<class "SecMirror.lvclass">)  [unwired: 7 in]
          n1785 = Subtract(x=w4988, y=w4987) -> (x-y=w4986:i32)
          n1786 = Absolute Value(x=w4986) -> (abs(x)=w4985:i32)
          n1787 = call-dynamic "Read State Machine.vi"("error in (no error)"=w4989, "Device in"=w4992) -> ("error out"=w5002:errorcluster, "State Machine.lvclass"=w5005:refnum<class "State Machine.lvclass">, "Device out"=w5015:refnum<class "SecMirror.lvclass">)  [unwired: 7 in]
          n1788 = To Unsigned Long Integer(number=w4985) -> (unsigned 32bit integer=w4982:u32)
          n1789 = Add(x=w4982, y=u32 25000 ("period")) -> (x+y=w4983:u32)
          n1790 = call-dynamic "Verif Clock 2.vi"("error in (no error)"=w5002, "period (ms)"=w4983, "State Machine in"=w5005) -> ("error out"=w5001:errorcluster, "time elapsed"=→"time elapsed 2":u32, "State Machine out"=w5004:refnum<class "State Machine.lvclass">)  [unwired: 6 in]
          n1791 = call-dynamic "Read Timeout 2.vi"("error in (no error)"=w5001, "State Machine in"=w5004) -> ("error out"=w5000:errorcluster, "Timeout 2"=w4978:bool, "State Machine out"=w5003:refnum<class "State Machine.lvclass">)  [unwired: 7 in]
          n1792 = call-dynamic "Read State.vi"("error in (no error)"=w5000, "State Machine in"=w5003) -> ("error out"=w5010:errorcluster, "State"=w4981:i32, "State Machine out"=w5011:refnum<class "State Machine.lvclass">)  [unwired: 7 in]
          n1793 = Equal To 0?(x=w4981) -> (x = 0?=w4976:bool)
          n1794 = Equal?(x=w4981, y=90) -> (x = y?=w4979:bool)
          n1795 = call-dynamic "Write State Machine.vi"("error in (no error)"=w5010, "State Machine.lvclass"=w5011, "Device in"=w5015) -> ("error out"=w5014:errorcluster, "Device out"=w5016:refnum<class "SecMirror.lvclass">)  [unwired: 7 in]
          n1796 = call-dynamic "Write SecMirror.lvclass.vi"("error in (no error)"=w5014, "SecMirror.lvclass"=w5016, "TelFocus in"=w5021) -> ("error out"=w5018:errorcluster, "TelFocus out"=w5020:refnum<class "TelFocus.lvclass">)  [unwired: 7 in]
          n1797 = Or(x=w4979, y=w4978) -> (x .or. y?=w4977:bool)
          n1798 = call-dynamic "Write TelFocus.lvclass.vi"("error in (no error)"=w5018, "TelFocus.lvclass"=w5020, "S4GUI in"=w5019) -> ("error out"=w5007:errorcluster, "S4GUI out"=w4999:refnum<class "S4GUI.lvclass">)  [unwired: 7 in]
          n1799 = case shown="False" w4977 {
            tunnel: w5006 -> [w5026 _]
            tunnel: [w5026 u32 1 ("Obs_state")] -> w4996
            tunnel: w4999 -> [w5025 w5031]
            tunnel: [w5025 w5030] -> w4998
            tunnel: [w5024 FALSE] -> w4975
            tunnel: w4976 -> [w5024 _]
            frame False {
            }
            frame True {
              n1800 = Bundle By Name(cluster=w5031, "Error Msg"="ERROR: moving telescope focus timeout  (S4GUI:HandleObservationSync.vi - state 361)") -> (w5030:refnum<class "S4GUI.lvclass">)
            }
          }
          n1801 = Increment(x=w4996) -> (x+1=w4995:u32)
          n1802 = Select(t=w4995, s=w4975, f=w4996) -> (s? t:f=w5009:u32)
          n1803 = Bundle By Name(cluster=w4998, "Obs_state"=w5009) -> (w5008:refnum<class "S4GUI.lvclass">)
        }
        frame 362 {
          # "Envia dados para o header das imagens (Channel:Run.vi - estado 58)"
          n1804 = call-dynamic "Read AcquisitionA.vi"("error in (no error)"=w5077, "S4ACS_GUI in"=w5078) -> ("error out"=w5054:errorcluster, "Acquisition.lvclass"=w5057:refnum<class "Acquisition.lvclass">, "S4ACS_GUI out"=w5080:refnum<class "S4GUI.lvclass">)  [unwired: 7 in]
          n1805 = call-dynamic "Read enabled.vi"("error in (no error)"=w5054, "Server in"=w5057) -> ("error out"=w5053:errorcluster, "enabled"=w5055:bool, "Server out"=w5056:refnum<class "Acquisition.lvclass">)  [unwired: 7 in]
          n1806 = case shown="True" w5055 {
            tunnel: w5056 -> [w5136 w5151]
            tunnel: w5053 -> [w5135 w5150]
            tunnel: [w5136 w5148] -> w5081
            tunnel: [w5135 w5147] -> w5079
            frame False {
            }
            frame True {
              n1807 = call-dynamic "Read Channel.vi"("error in (no error)"=w5150, "Acquisition in"=w5151) -> ("error out"=w5143:errorcluster, "Channel.lvclass"=w5142:refnum<class "Channel.lvclass">, "Acquisition out"=w5149:refnum<class "Acquisition.lvclass">)  [unwired: 7 in]
              n1808 = call-dynamic "Read State Machine.vi"("error in (no error)"=w5143, "Device in"=w5142) -> ("error out"=w5144:errorcluster, "State Machine.lvclass"=w5146:refnum<class "State Machine.lvclass">, "Device out"=w5140:refnum<class "Channel.lvclass">)  [unwired: 7 in]
              n1809 = call "Next State.vi"("error in (no error)"=w5144, "New_State"=58, "State Machine in"=w5146) -> ("error out"=w5137:errorcluster, "State Machine out"=w5138:refnum<class "State Machine.lvclass">)  [unwired: 7 in]
              n1810 = call-dynamic "Write State Machine.vi"("error in (no error)"=w5137, "State Machine.lvclass"=w5138, "Device in"=w5140) -> ("error out"=w5139:errorcluster, "Device out"=w5141:refnum<class "Channel.lvclass">)  [unwired: 7 in]
              n1811 = call-dynamic "Write Channel.vi"("error in (no error)"=w5139, "Channel.lvclass"=w5141, "Acquisition in"=w5149) -> ("error out"=w5147:errorcluster, "Acquisition out"=w5148:refnum<class "Acquisition.lvclass">)  [unwired: 7 in]
            }
          }
          n1812 = call-dynamic "Write AcquisitionA.vi"("error in (no error)"=w5079, "Acquisition.lvclass"=w5081, "S4ACS_GUI in"=w5080) -> ("error out"=w5072:errorcluster, "S4ACS_GUI out"=w5073:refnum<class "S4GUI.lvclass">)  [unwired: 7 in]
          n1813 = call "Read AcquisitionB.vi"("error in (no error)"=w5072, "S4ACS_GUI in"=w5073) -> ("error out"=w5050:errorcluster, "Acquisition.lvclass"=w5052:refnum<class "Acquisition.lvclass">, "S4ACS_GUI out"=w5070:refnum<class "S4GUI.lvclass">)  [unwired: 7 in]
          n1814 = call-dynamic "Read enabled.vi"("error in (no error)"=w5050, "Server in"=w5052) -> ("error out"=w5049:errorcluster, "enabled"=w5048:bool, "Server out"=w5051:refnum<class "Acquisition.lvclass">)  [unwired: 7 in]
          n1815 = case shown="True" w5048 {
            tunnel: w5051 -> [w5119 w5134]
            tunnel: w5049 -> [w5118 w5133]
            tunnel: [w5119 w5131] -> w5071
            tunnel: [w5118 w5130] -> w5069
            frame False {
            }
            frame True {
              n1816 = call-dynamic "Read Channel.vi"("error in (no error)"=w5133, "Acquisition in"=w5134) -> ("error out"=w5126:errorcluster, "Channel.lvclass"=w5125:refnum<class "Channel.lvclass">, "Acquisition out"=w5132:refnum<class "Acquisition.lvclass">)  [unwired: 7 in]
              n1817 = call-dynamic "Read State Machine.vi"("error in (no error)"=w5126, "Device in"=w5125) -> ("error out"=w5127:errorcluster, "State Machine.lvclass"=w5129:refnum<class "State Machine.lvclass">, "Device out"=w5123:refnum<class "Channel.lvclass">)  [unwired: 7 in]
              n1818 = call "Next State.vi"("error in (no error)"=w5127, "New_State"=58, "State Machine in"=w5129) -> ("error out"=w5120:errorcluster, "State Machine out"=w5121:refnum<class "State Machine.lvclass">)  [unwired: 7 in]
              n1819 = call-dynamic "Write State Machine.vi"("error in (no error)"=w5120, "State Machine.lvclass"=w5121, "Device in"=w5123) -> ("error out"=w5122:errorcluster, "Device out"=w5124:refnum<class "Channel.lvclass">)  [unwired: 7 in]
              n1820 = call-dynamic "Write Channel.vi"("error in (no error)"=w5122, "Channel.lvclass"=w5124, "Acquisition in"=w5132) -> ("error out"=w5130:errorcluster, "Acquisition out"=w5131:refnum<class "Acquisition.lvclass">)  [unwired: 7 in]
            }
          }
          n1821 = call "Write AcquisitionB.vi"("error in (no error)"=w5069, "Acquisition.lvclass"=w5071, "S4ACS_GUI in"=w5070) -> ("error out"=w5065:errorcluster, "S4ACS_GUI out"=w5064:refnum<class "S4GUI.lvclass">)  [unwired: 7 in]
          n1822 = call-dynamic "Read AcquisitionC.vi"("error in (no error)"=w5065, "S4ACS_GUI in"=w5064) -> ("error out"=w5045:errorcluster, "Acquisition.lvclass"=w5047:refnum<class "Acquisition.lvclass">, "S4ACS_GUI out"=w5067:refnum<class "S4GUI.lvclass">)  [unwired: 7 in]
